vi "Set Properties.vi"(5 "rampDown":dbl, 6 "transition":dbl, 7 "rampUp":dbl, 8 "profile":u16, 9 "systemTimingModel":i64, 10 "sampleRate":dbl=51200.0, 11 "RefIn":u32) -> (2 "error out":errorcluster, 3 "refOut":u32)   [LabVIEW 2021]
uses:
  <vilib>/addons/_NISVFA/_Generation/Signal Generation/SV Signal/sv_System Timing Model.ctl
  <vilib>/addons/_NISVFA/_Generation/Signal Generation/SV Sinusoid/SV Sinusoid.lvclass
  C:/Program Files/National Instruments/LabVIEW 2021/vi.lib/addons/_NISVFA/_Generation/Signal Generation/SV Signal/SV Signal.lvclass
  <vilib>/addons/_NISVFA/_Generation/Signal Generation/SV Signal/Write Sample Rate.vi
  <vilib>/addons/_NISVFA/_Generation/Signal Generation/SV Signal/Write System Timing Model.vi
  <vilib>/addons/_NISVFA/_Generation/Signal Generation/SV Signal/Write Ramp Parameters.vi
  <vilib>/addons/_NISVFA/_Generation/Signal Generation/SV Signal/SV Signal.lvclass
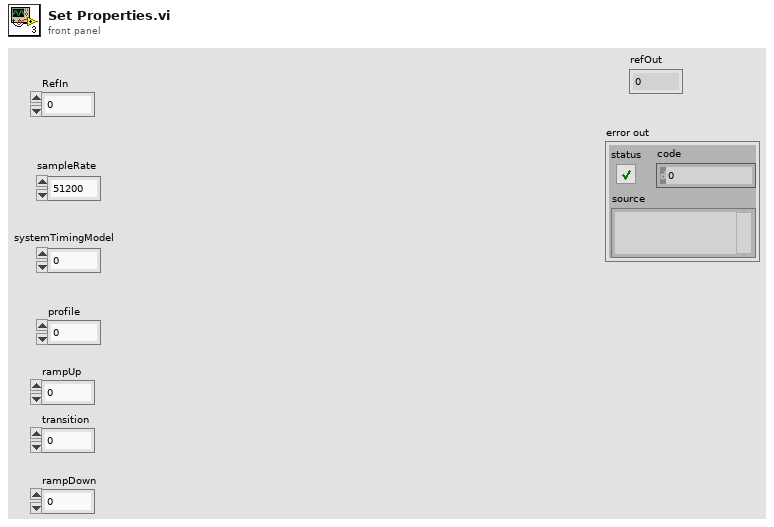
[diagram p1: front panel]
types:
  T1 = cluster{"profile":enum16{"Linear", "Half cosine"}, "durations [s]":cluster{"ramp-up":dbl, "transition":dbl, "ramp-down":dbl}}
  T2 = typedef "SV Signal.lvclass/sv_System Timing Model.ctl" = i64
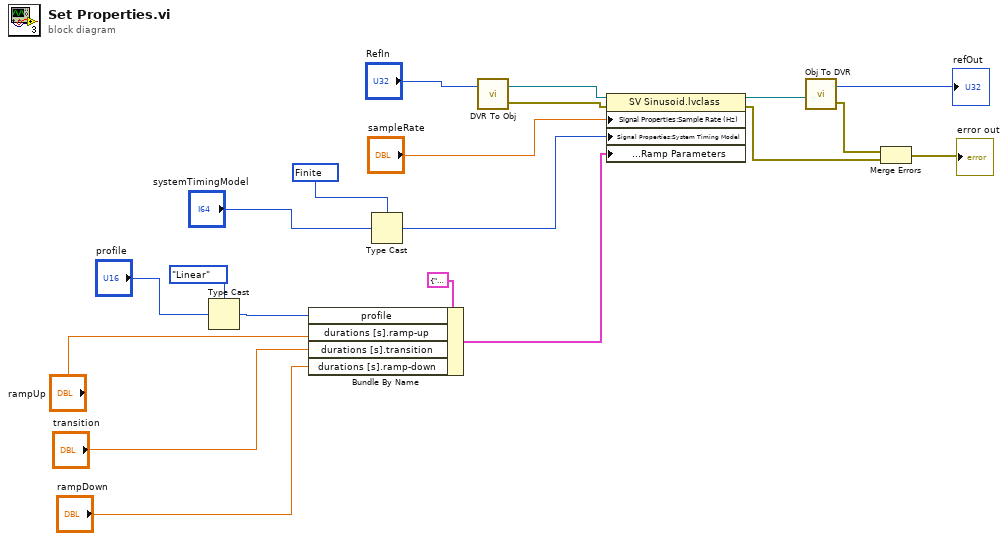
[diagram p0: block diagram]
diagram:
  w10 = T2 10178 items=["Finite"=10178, "-"=-1, "Continuous"=10123, "-"=-2, "Settled"=110123, "Averaged"=210123, "Discrete Sweep"=310123, "Continuous Sweep"=410123] ("System Timing Model")
  n1 = Type Cast(type=enum16{"Linear", "Half cosine"}."Linear" ("profile"), x="profile") -> (*(type *) &x=w5:enum16{"Linear", "Half cosine"})
  n2 = Bundle By Name(cluster=T1 {"profile"=enum."Linear", "durations [s]"={"ramp-up"=0.0, "transition"=0.0, "ramp-down"=0.0}} ("rampParameter"), "profile"=w5, "durations [s].ramp-up"="rampUp", "durations [s].transition"="transition", "durations [s].ramp-down"="rampDown") -> (w7:T1)
  n3 = Type Cast(type=w10, x="systemTimingModel") -> (*(type *) &x=w9:T2)
  n4 = call "DVR To Obj.vi"("RefIn"="RefIn") -> ("error_out"=w19:errorcluster, "data"=w20:refnum<class "SV Sinusoid.lvclass">)  [unwired: 1 in]
  n5 = property class="SV Sinusoid.lvclass"(reference=w20, error in=w19, "Signal Properties:Sample Rate (Hz)"="sampleRate", "Signal Properties:System Timing Model"=w9, "Signal Properties:Ramps:Ramp Parameters"=w7) -> (reference out=w16:refnum<class "SV Sinusoid.lvclass">, error out=w15:errorcluster)
  n6 = call "Obj To DVR.vi"("signal configuration"=w16) -> ("error_out"=w14:errorcluster, "dataValueReference"=→"refOut":u32)  [unwired: 1 in]
  n7 = Merge Errors(w14, w15) -> (→"error out":errorcluster)
